vi "NET-RX Spawn UDP Service.vi"(5 "Max Rx Byte Size":i32=10000, 7 "Module ID":i32=-1, 8 "error in":errorcluster, 9 "Caller MsgQ":refnum<class "DQMH-GenNet Message Queue.lvclass">, 10 "Stop Module":refnum<user-event>, 11 "UDP Connection ID":refnum<k16>) -> (0 "error out":errorcluster)   [LabVIEW 2020, in "GenNet-Client.lvlib"]
doc: "____\nHAMPEL SOFTWARE ENGINEERING v3.8.0 (2023-12-18 14:41)"
uses:
  GenNet-Client.lvlib
  GenNet-Server/Stop Argument--cluster.ctl
  DQMH-GenNet Message Queue.lvclass
  NET-RX UDP Service.vi
  GenNet-Server/GenNet-Server.lvlib
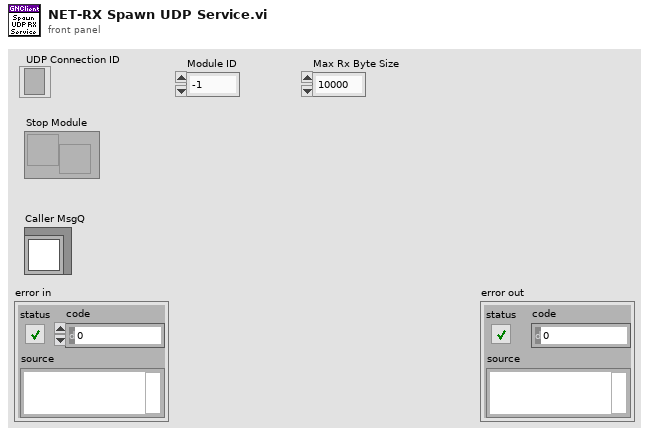
[diagram p1: front panel]
types:
  T1 = enum32{"Invalid", "Standard", "Closed", "Hidden", "Minimized", "Maximized"}
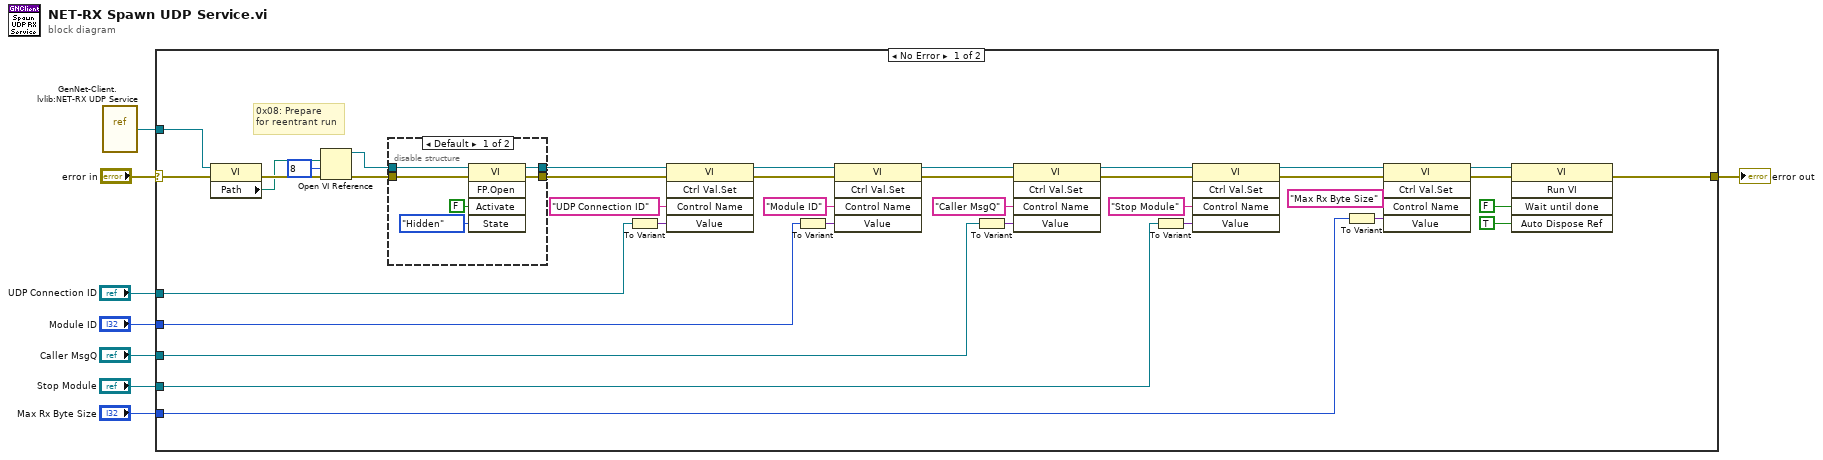
[diagram p0: block diagram]
diagram:
  n1 = vi-ref "GenNet-Client.lvlib:NET-RX UDP Service.vi"() -> (w2:refnum<vi>)
  n2 = case shown="No Error" "error in" {
    selector: "error in" -> [w19 w54]
    tunnel: [w18 w54] -> w4
    tunnel: "Caller MsgQ" -> [w26 _]
    tunnel: "Module ID" -> [w25 _]
    tunnel: w2 -> [w24 _]
    tunnel: "UDP Connection ID" -> [w23 _]
    tunnel: "Stop Module" -> [w20 _]
    tunnel: "Max Rx Byte Size" -> [w9 _]
    frame No Error {
      # "0x08: Prepare \nfor reentrant run"
      n3 = property class="VI"(reference=w24, error in=w19) -> (error out=w38:errorcluster, "Path"=w37:path)  [unwired: 1 out]
      n4 = Open VI Reference(vi path=w37, options=8, error in (no error)=w38) -> (vi reference=w40:refnum<vi>, error out=w41:errorcluster)  [unwired: 3 in]
      n5 = disable-structure shown="Default" {
        disable-tunnel: [w51 w53] -> w36
        disable-tunnel: w41 -> [w50 w52]
        disable-tunnel: [w49 w52] -> w35
        disable-tunnel: w40 -> [w48 w53]
        frame condition #0 (active) {
          n6 = invoke class="VI" method="FP.Open"(reference=w48, error in=w50, "Activate"=FALSE ("Activate?"), "State"=T1."Hidden") -> (reference out=w51:refnum<vi>, error out=w49:errorcluster)  [unwired: 1 in, 3 out]
        }
        frame condition #1 {
        }
      }
      n7 = To Variant(anything=w23) -> (Variant=w42:variant)
      n8 = invoke class="VI" method="Ctrl Val.Set"(reference=w36, error in=w35, "Control Name"="UDP Connection ID", "Value"=w42) -> (reference out=w31:refnum<vi>, error out=w30:errorcluster)  [unwired: 1 in, 3 out]
      n9 = To Variant(anything=w25) -> (Variant=w33:variant)
      n10 = invoke class="VI" method="Ctrl Val.Set"(reference=w31, error in=w30, "Control Name"="Module ID", "Value"=w33) -> (reference out=w29:refnum<vi>, error out=w28:errorcluster)  [unwired: 1 in, 3 out]
      n11 = To Variant(anything=w26) -> (Variant=w27:variant)
      n12 = invoke class="VI" method="Ctrl Val.Set"(reference=w29, error in=w28, "Control Name"="Caller MsgQ", "Value"=w27) -> (reference out=w16:refnum<vi>, error out=w13:errorcluster)  [unwired: 1 in, 3 out]
      n13 = To Variant(anything=w20) -> (Variant=w22:variant)
      n14 = invoke class="VI" method="Ctrl Val.Set"(reference=w16, error in=w13, "Control Name"="Stop Module", "Value"=w22) -> (reference out=w15:refnum<vi>, error out=w12:errorcluster)  [unwired: 1 in, 3 out]
      n15 = To Variant(anything=w9) -> (Variant=w17:variant)
      n16 = invoke class="VI" method="Ctrl Val.Set"(reference=w15, error in=w12, "Control Name"="Max Rx Byte Size", "Value"=w17) -> (reference out=w14:refnum<vi>, error out=w11:errorcluster)  [unwired: 1 in, 3 out]
      n17 = invoke class="VI" method="Run VI"(reference=w14, error in=w11, "Wait until done"=FALSE ("Wait Until Done"), "Auto Dispose Ref"=TRUE ("Auto Dispose Reference")) -> (error out=w18:errorcluster)  [unwired: 1 in, 4 out]
    }
    frame Error {
    }
  }
  "error out" <- w4
